vi "NewPyTool.vi"(8 "error in (no error)":errorcluster, 10 "Description":string, 11 "Name":string) -> (0 "error out":errorcluster, 3 "PyTool out":refnum<class "PyTool.lvclass">)   [LabVIEW 2025, in "Tools.lvlib" / "PyTool.lvclass"]
uses:
  PyTool.lvclass
  PyTool.lvclass/PyTool.ctl
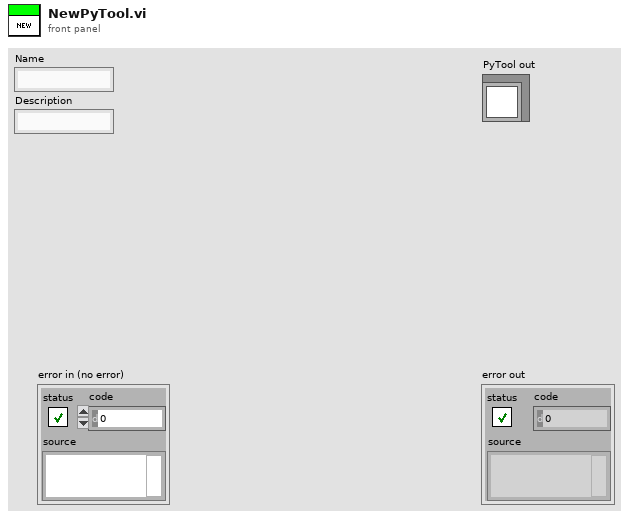
[diagram p1: front panel]
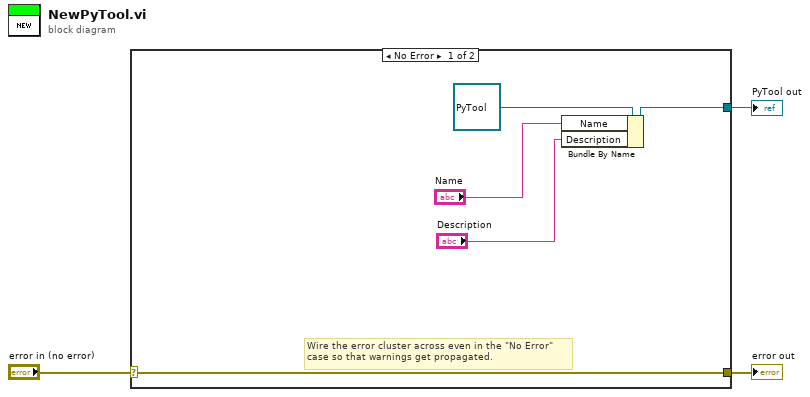
[diagram p0: block diagram]
diagram:
  n1 = case shown="No Error" "error in (no error)" {
    selector: "error in (no error)" -> [w8 w9]
    tunnel: [w8 w9] -> w2
    tunnel: [w6 _] -> w1
    frame No Error {
      # "Wire the error cluster across even in the \"No Error\"\ncase so that warnings get propagated."
      n2 = Bundle By Name(cluster=refnum<class "PyTool.lvclass"> refnum ("PyTool out"), "Name"="Name", "Description"="Description") -> (w6:refnum<class "PyTool.lvclass">)
    }
    frame Error {
    }
  }
  "error out" <- w2
  "PyTool out" <- w1
